vi "HowForebrainPerception.vi"() -> (4 "BatteryGauge":dbl)   [LabVIEW 2010]
doc: "This SubVI takes clean How sense data from the Midbrain and layers perception onto it to be passed to the THINK processes in the Forebrain"
uses:
  6-OCU Neurons/CommonIndicators.ctl
  5.0-Global.vi
  <vilib>/ptbypt/NI_PtbyPt.lvlib
panel:
  # "This SubVI adds \nperception onto the\nHow data comming\nfrom the Midbrain"
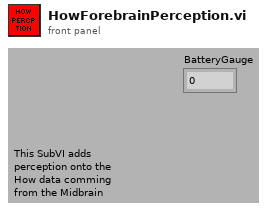
[diagram p1: front panel]
types:
  T1 = typedef "CommonIndicators.ctl" = cluster{"Speed":dbl, " Heading":cluster{dbl, dbl}, "MissionTime":dbl, "Battery":dbl, "MAP":bool, "LIDAR":bool, "ManualMissionMap":picture, "ManualModeLIDAR":picture, "ManualModeStop":bool, "How?":bool, "Where?":bool, "What?":bool, "ActManual":bool, "CollisionLight ":bool, "Ready":bool}
  T2 = cluster{"X (Current)":dbl, "Y (Current) ":dbl, "Heading":dbl, "Steering Angle":dbl}
  T3 = typedef "How Sensor Typedef.ctl" = cluster{"Motor Speed Integer":i32, "Drive Position Integer":i32, "Lidar Position Integer":i32, "Lidar Motor Position Integer":i32, "Steering Position Integer":i32, "Battery Voltage Fxp":dbl, "Drive Encoder Cable Check":bool, "Lidar Drive Encoder Cable Check":bool, "Steer Encoder Cable Check":bool, "Lidar Pos Encoder Cable Check":bool, "Mod Buttons & Blinky Cable Check":bool, "Lidar Data Cable Check":bool, "Drive Motor Cable Check":bool, "Vector Nav Cable Check":bool, "Lidar Drive Cable Check":bool, "Steer Drive Cable Check":bool, "Reverse?":bool, "2.1  Steering Control Voltage":dbl, "2.1 Drive Control Voltage":dbl, "2.1  Lidar Control Voltage":dbl, "2.5.7 A*B":dbl, "2.1  Steering PID Output":dbl, "2.1 Drive PID Output":dbl, "2.1  Lidar PID Output":dbl, "2.1.1 Drive Error":dbl, "2.1.1 Drive Error I":dbl, "2.1.1 Drive Error D":dbl, "2.1.2 Steering Error":dbl, "2.1.2 Steering Error I":dbl, "2.1.2 Steering Error D":dbl, "2.1.3 Lidar Error":dbl, "2.1.3 Lidar Error I":dbl, "2.1.3 Lidar Error D":dbl, "VectorNav Ack Query":bool, "VectorNav Read Byte":u8, "VectorNav Read Status":enum16{"Waiting", "Reading", "Done"}}
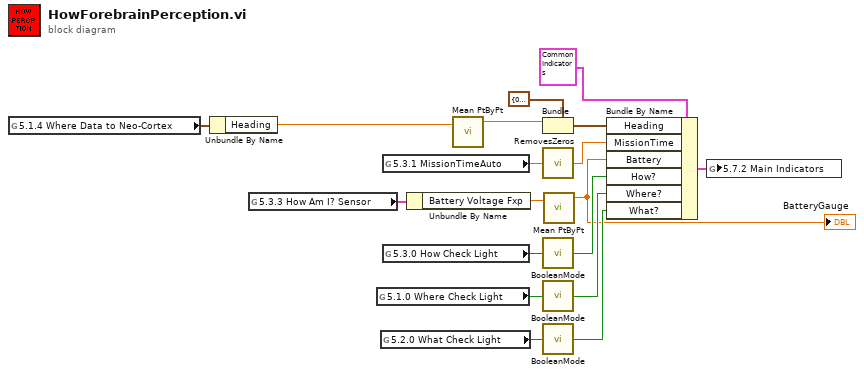
[diagram p0: block diagram]
diagram:
  n1 = global read "5.0-Global.vi" "5.1.4 Where Data to Neo-Cortex"() -> (w16:T2)
  n2 = Unbundle By Name(w16) -> ("Heading"=w13:dbl)
  n3 = global read "5.0-Global.vi" "5.3.3 How Am I? Sensor"() -> (w12:T3)
  n4 = global read "5.0-Global.vi" "5.1.0 Where Check Light"() -> (w8:bool)
  n5 = global read "5.0-Global.vi" "5.2.0 What Check Light"() -> (w6:bool)
  n6 = global read "5.0-Global.vi" "5.3.1 MissionTimeAuto"() -> (w4:dbl)
  n7 = global read "5.0-Global.vi" "5.3.0 How Check Light"() -> (w10:bool)
  n8 = Unbundle By Name(w12) -> ("Battery Voltage Fxp"=w11:dbl)
  n9 = call <vilib>:"Mean PtByPt.vi"("x"=w13) -> ("mean"=w1:dbl)  [unwired: 3 in, 1 out]
  n10 = Bundle(cluster=cluster{dbl, dbl} {0.0, 0.0} ("Heading"), w1) -> (w15:cluster{dbl, dbl})  [unwired: 1 in]
  n11 = call "RemovesZeros.vi"("5.3.1 MissionTimeAuto 2"=w4) -> ("5.3.1 MissionTimeAuto"=w3:dbl)
  n12 = call "BooleanMode.vi"("5.3.0 How Check Light  2"=w10) -> ("5.3.0 How Check Light"=w9:bool)
  n13 = call "BooleanMode.vi"("5.3.0 How Check Light  2"=w8) -> ("5.3.0 How Check Light"=w7:bool)
  n14 = call "BooleanMode.vi"("5.3.0 How Check Light  2"=w6) -> ("5.3.0 How Check Light"=w5:bool)
  n15 = call <vilib>:"Mean PtByPt.vi"("x"=w11) -> ("mean"=w2:dbl)  [unwired: 3 in, 1 out]
  "BatteryGauge" <- w2
  n16 = Bundle By Name(cluster=T1 {"Speed"=0.0, " Heading"={0.0, 34.390870865624734}, "MissionTime"=0.0, "Battery"=0.0, "MAP"=FALSE, "LIDAR"=FALSE, "ManualMissionMap"=bytes[0], "ManualModeLIDAR"=bytes[0], "ManualModeStop"=FALSE, "How?"=FALSE, "Where?"=FALSE, "What?"=FALSE, "ActManual"=FALSE, "CollisionLight "=FALSE, "Ready"=FALSE} ("5.7.2 Main Indicators"), "Heading"=w15, "MissionTime"=w3, "Battery"=w2, "How?"=w9, "Where?"=w7, "What?"=w5) -> (w18:T1)
  n17 = global write "5.0-Global.vi" "5.7.2 Main Indicators"(w18) -> ()
